vi "UnDecorator.vi"(8 "error in (no error)":errorcluster, 11 "DataVer3 in":refnum<class "DataVer3.lvclass">) -> (0 "error out":errorcluster, 2 "DecoratorData Out":refnum<class "Data.lvclass">, 3 "DataVer3 out":refnum<class "DataVer3.lvclass">)   [LabVIEW 2013, in "DataVer3.lvclass"]
uses:
  DataVer3.lvclass
  Data.lvclass/Data.lvclass
  DataVer3.lvclass/DataVer3.ctl
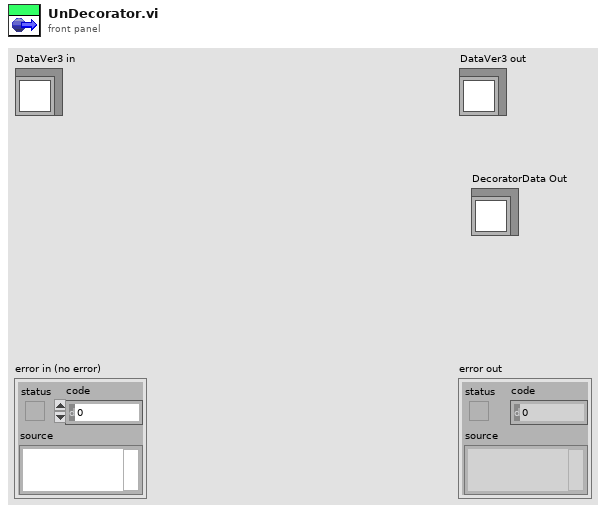
[diagram p1: front panel]
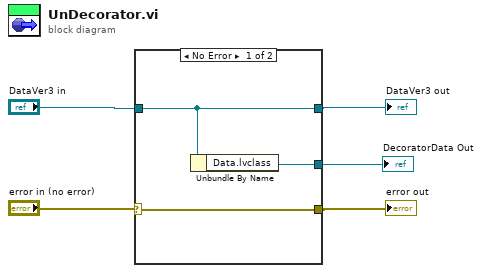
[diagram p0: block diagram]
diagram:
  n1 = case shown="No Error" "error in (no error)" {
    selector: "error in (no error)" -> [w8 w10]
    tunnel: [w8 w10] -> w3
    tunnel: [w7 w9] -> w4
    tunnel: "DataVer3 in" -> [w7 w9]
    tunnel: [w6 _] -> w1
    frame No Error {
      n2 = Unbundle By Name(w7) -> ("Data.lvclass"=w6:refnum<class "Data.lvclass">)
    }
    frame Error {
    }
  }
  "error out" <- w3
  "DataVer3 out" <- w4
  "DecoratorData Out" <- w1
